vi "OPC UA Write.vi"() -> ()   [LabVIEW 2023]
uses:
  <vilib>/OPCUA/controls/NodeId.ctl
  <vilib>/OPCUA/controls/Write Status.ctl
  <vilib>/OPCUA/client/Multiple Write Variant.vi
  <vilib>/OPCUA/NI OPC UA Client.lvlib
panel:
  in  "Temp reading mode":bool
  in  "Temperature Value":dbl
  in  "Node ID":string
  in  "stop":bool
  in  "server endpoint URL":string
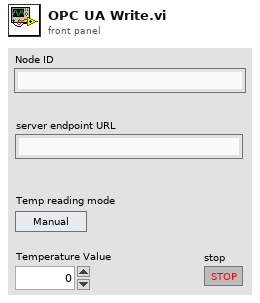
[diagram p1: front panel]
types:
  T1 = cluster{"message mode":enum16{"None", "Sign", "Sign and Encrypt"}, "security":enum16{"Basic256", "Basic128Rsa15"}}
  T2 = typedef "OPC UA Client Refnum.ctl" = refnum<k21>
  T3 = typedef "NodeId.ctl" = string
  T4 = typedef "Write Status.ctl" = u32
  T5 = cluster{"node ID":T3, "value":dbl, "timestamp (current time)":timestamp, "node status":T4}
  T6 = cluster{"node ID":T3, "value":dbl, "timestamp (current time)":timestamp, "node status":T4}[]
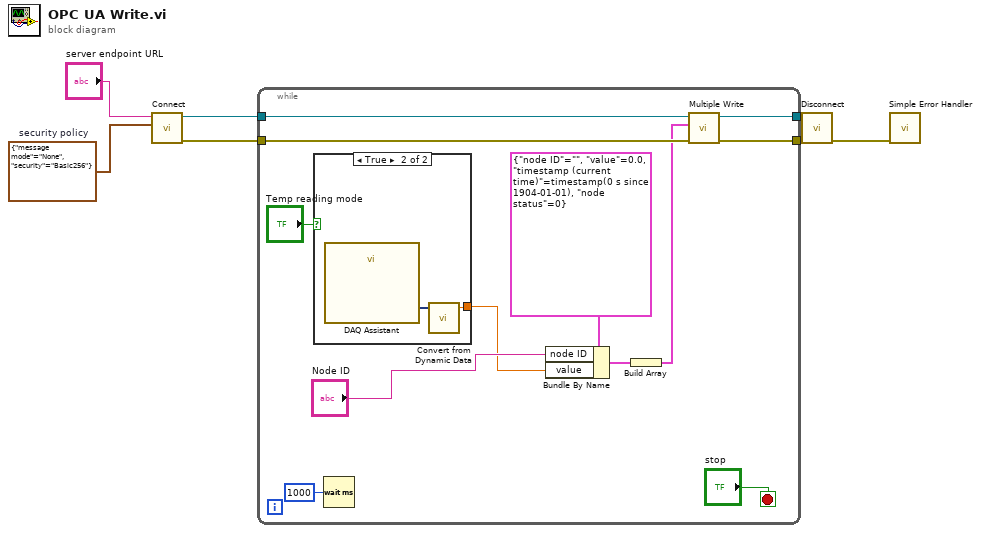
[diagram p0: block diagram]
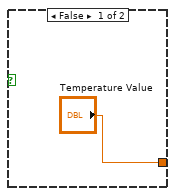
[diagram p2: hidden frame]
diagram:
  w1 = T1 {"message mode"=enum."None", "security"=enum."Basic256"}  # security policy
  n1 = call <vilib>:"Connect.vi"("security policy"=w1, "server endpoint URL"="server endpoint URL") -> ("error out"=w6:errorcluster, "OPC UA client refnum out"=w4:T2)  [unwired: 7 in, 1 out]
  n2 = while {
    tunnel: w6 -> [w17]
    tunnel: [w16] -> w5
    tunnel: w4 -> [w15]
    tunnel: [w14] -> w3
    stop <- "stop" stop-if-true
    n3 = case shown="True" "Temp reading mode" {
      tunnel: ["Temperature Value" w21] -> w9
      frame False {
      }
      frame True {
        n4 = call "DAQ Assistant"() -> ("data"=w22:dynamicdata)  [unwired: 17 in, 2 out]
        n5 = call "Convert from Dynamic Data"("Dynamic Data Type"=w22) -> ("Scalar"=w21:dbl)  [unwired: 3 in]
      }
    }
    n6 = Wait (ms)(milliseconds to wait=u32 1000) -> ()  [unwired: 1 out]
    n7 = Bundle By Name(cluster=T5 {"node ID"="", "value"=0.0, "timestamp (current time)"=timestamp(0 s since 1904-01-01), "node status"=0} ("request"), "node ID"="Node ID", "value"=w9) -> (w13:T5)
    n8 = Build Array(w13) -> (w11:T6)
    n9 = call-poly <vilib>:"Multiple Write.vi"("error in (no error)"=w17, "requests"=w11, "OPC UA client refnum in"=w15) -> ("error out"=w16:errorcluster, "OPC UA client refnum out"=w14:T2)  [unwired: 5 in, 2 out]
  }
  n10 = call <vilib>:"Disconnect.vi"("error in (no error)"=w5, "OPC UA client refnum in"=w3) -> ("error out"=w7:errorcluster)  [unwired: 9 in]
  n11 = call <vilib>:"Simple Error Handler.vi"("error in (no error)"=w7) -> ()  [unwired: 4 in, 5 out]
